vi "Polling Start Stop.vi"(8 "Error In":errorcluster, 10 "Start Polling":bool, 11 "CS++BaseActor in":refnum<class "CS++BaseActor.lvclass">) -> (0 "Error Out":errorcluster, 3 "CS++BaseActor out":refnum<class "CS++BaseActor.lvclass">)   [LabVIEW 2015, in "CS++BaseActor.lvlib" / "CS++BaseActor.lvclass"]
doc: "Start or stop polling."
uses:
  CS++BaseActor.lvclass
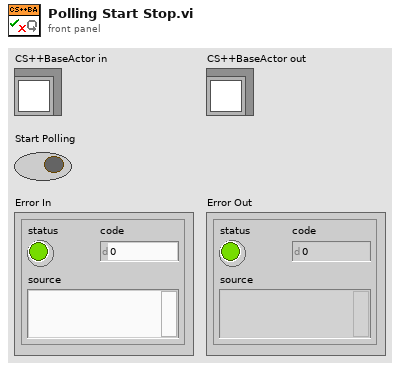
[diagram p1: front panel]
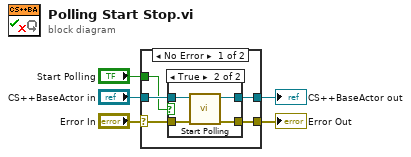
[diagram p0: block diagram]
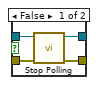
[diagram p2: hidden frame]
diagram:
  n1 = case shown="No Error" "Error In" {
    selector: "Error In" -> [w8 w20]
    tunnel: [w7 w20] -> w4
    tunnel: [w9 w19] -> w2
    tunnel: "CS++BaseActor in" -> [w10 w19]
    tunnel: "Start Polling" -> [w6 _]
    frame No Error {
      n2 = case shown="True" w6 {
        tunnel: w10 -> [w14 w18]
        tunnel: [w11 w17] -> w9
        tunnel: w8 -> [w13 w16]
        tunnel: [w12 w15] -> w7
        frame False {
          n3 = call "Stop Polling.vi"("Error In"=w13, "CS++BaseActor in"=w14) -> ("Error Out"=w12:errorcluster, "CS++BaseActor out"=w11:refnum<class "CS++BaseActor.lvclass">)  [unwired: 8 in]
        }
        frame True {
          n4 = call "Start Polling.vi"("Error In"=w16, "CS++BaseActor in"=w18) -> ("Error Out"=w15:errorcluster, "CS++BaseActor out"=w17:refnum<class "CS++BaseActor.lvclass">)  [unwired: 8 in]
        }
      }
    }
    frame Error {
    }
  }
  "Error Out" <- w4
  "CS++BaseActor out" <- w2
